vi "Set Panel Initial State.vi"(10 "Title":string, 11 "Main Vi Ref":refnum<vi>) -> (0 "error out":errorcluster)   [LabVIEW 2021, in "Panther Dashboard.lvlib"]
uses:
  Panther Dashboard.lvlib
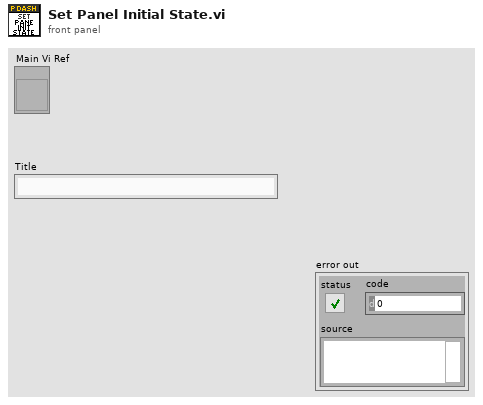
[diagram p1: front panel]
types:
  T1 = enum32{"Invalid", "Standard", "Closed", "Hidden", "Minimized", "Maximized"}
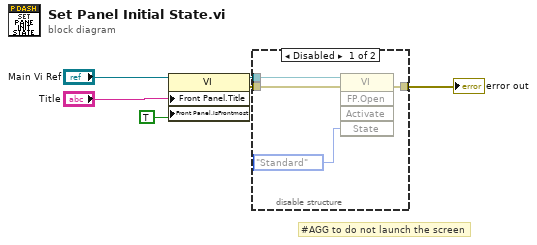
[diagram p0: block diagram]
diagram:
  # "#AGG to do not launch the screen"
  n1 = property on="Property Node" class="VI"(reference="Main Vi Ref", "Front Panel.Title"="Title", "Front Panel.IsFrontmost"=TRUE ("Front Panel Window:Is Frontmost")) -> (reference out=w2:refnum<vi>, error out=w6:errorcluster)  [unwired: 1 in]
  n2 = disable-structure shown="Disabled" {
    disable-tunnel: w6 -> [w10 _]
    disable-tunnel: [w9 _] -> w5
    disable-tunnel: w2 -> [w7 _]
    frame Disabled {
      n3 = invoke on="Invoke Node" class="VI" method="FP.Open"(reference=w7, error in=w10, "State"=T1."Standard") -> (error out=w9:errorcluster)  [unwired: 2 in, 4 out]
    }
    frame Enabled {
    }
  }
  "error out" <- w5
